vi "fill_board.vi"(6 "Shape Report":T3(array[cluster]), 7 "Number pieces":i32, 9 "Replacement type":cluster{"Piece Type":T1, "Team Color":T2}, 10 "Dimensions":T4, 11 "Board Layout":cluster{"Piece Type":T1, "Team Color":T2}[][](array[cluster])) -> (3 "New Board Layout":cluster{"Piece Type":T1, "Team Color":T2}[][](array[cluster]))   [LabVIEW 2015]
uses:
  chess_piecetype_enum.ctl
  chess_teamcolor_enum.ctl
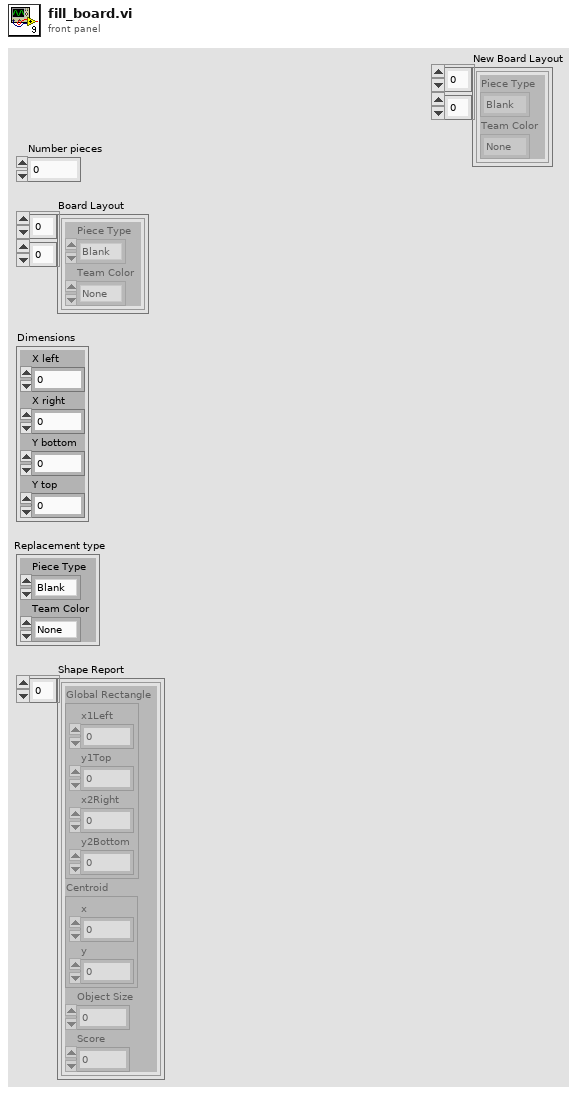
[diagram p1: front panel]
types:
  T1 = typedef "chess_piecetype_enum.ctl" = enum16{"Blank", "Pawn", "Rook", "Knight", "Bishop", "Queen", "King"}
  T2 = typedef "chess_teamcolor_enum.ctl" = enum16{"None", "Red", "Blue"}
  T3 = cluster{"Global Rectangle":cluster{"x1Left":i32, "y1Top":i32, "x2Right":i32, "y2Bottom":i32}, "Centroid":cluster{"x":sgl, "y":sgl}, "Object Size":u32, "Score":dbl}[]
  T4 = cluster{"X left":dbl, "X right":dbl, "Y bottom":dbl, "Y top":dbl}
  T5 = cluster{"Global Rectangle":cluster{"x1Left":i32, "y1Top":i32, "x2Right":i32, "y2Bottom":i32}, "Centroid":cluster{"x":sgl, "y":sgl}, "Object Size":u32, "Score":dbl}
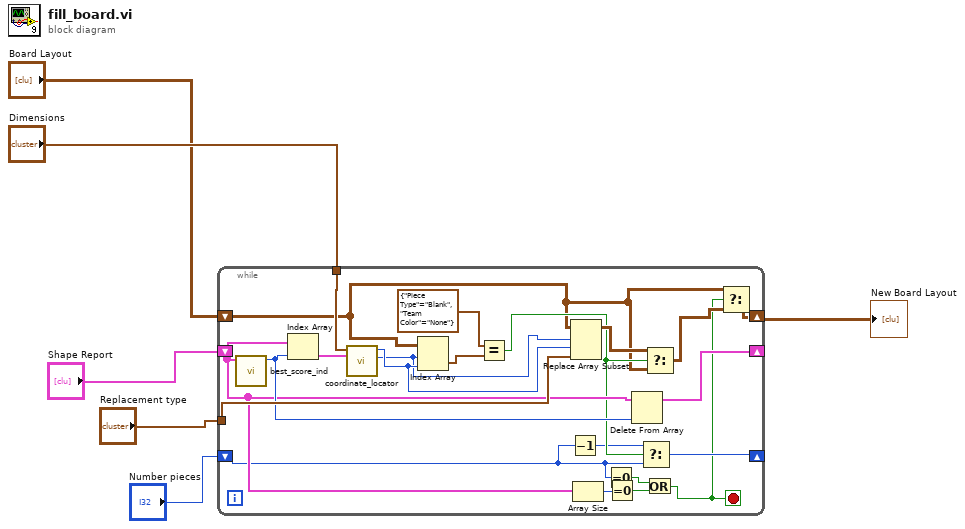
[diagram p0: block diagram]
diagram:
  n1 = while {
    tunnel: "Dimensions" -> [w27]
    tunnel: "Replacement type" -> [w22]
    shift-right: [w12] -> _
    shift-left: "Shape Report" -> [w19]
    shift-right: [w11] -> _
    shift-left: "Number pieces" -> [w15]
    shift-right: [w9] -> w2
    shift-left: "Board Layout" -> [w8]
    stop <- w7 stop-if-true
    n2 = call "best_score_ind.vi"("Shape Report"=w19) -> ("Max Ind"=w20:i32)  [unwired: 10 in]
    n3 = Index Array(array=w19, index=w20) -> (element=w28:T5)
    n4 = call "coordinate_locator.vi"("Shape Cluster"=w28, "Dimensions"=w27) -> ("y coord"=w23:i32, "x coord"=w24:i32)  [unwired: 8 in]
    n5 = Index Array(array=w8, index (row)=w23, index (col)=w24) -> (element=w26:cluster{"Piece Type":T1, "Team Color":T2})
    n6 = Equal?(x=cluster{"Piece Type":T1, "Team Color":T2} {"Piece Type"=enum."Blank", "Team Color"=enum."None"}, y=w26) -> (x = y?=w17:bool)
    n7 = Decrement(x=w15) -> (x-1=w16:i32)
    n8 = Replace Array Subset(array=w8, new element=w22, index (row)=w23, index (col)=w24) -> (w21:cluster{"Piece Type":T1, "Team Color":T2}[][])
    n9 = Array Size(array=w19) -> (size(s)=w18:i32)
    n10 = Equal To 0?(x=w15) -> (x = 0?=w14:bool)
    n11 = Equal To 0?(x=w18) -> (x = 0?=w13:bool)
    n12 = Delete From Array(array=w19, index=w20) -> (array with subset deleted=w12:T3)  [unwired: 1 in, 1 out]
    n13 = Select(t=w16, s=w17, f=w15) -> (s? t:f=w11:i32)
    n14 = Select(t=w21, s=w17, f=w8) -> (s? t:f=w10:cluster{"Piece Type":T1, "Team Color":T2}[][])
    n15 = Or(x=w14, y=w13) -> (x .or. y?=w7:bool)
    n16 = Select(t=w8, s=w7, f=w10) -> (s? t:f=w9:cluster{"Piece Type":T1, "Team Color":T2}[][])
  }
  "New Board Layout" <- w2
